vi "PicowattAVS47_Check_Queue.vi"(7 "error in (no error)":errorcluster caption="Fehler (Eingang, kein Fehler)", 10 "queue":refnum<queue>) -> (0 "error out":errorcluster caption="Fehler (Ausgang)", 1 "AVS47 Control Cluster":T1 {"AVS Excitation" items=["no Exc.", "3uV", "10uV", "30uV", "100uV", "300uV", "1mV", "3mV"]}, 3 "New Entries ?":bool)   [LabVIEW 2018]
uses:
  PicowattAVS47/AVS-Control-Cluster.ctl
panel:
  out "Numerisches Anzeigeelement":i32
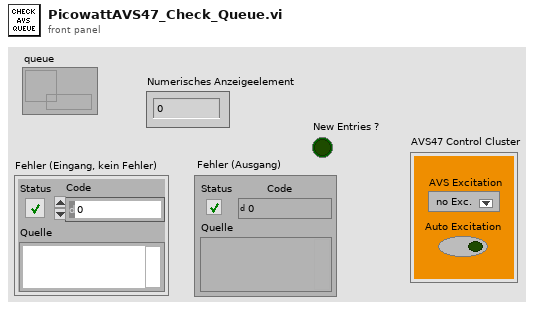
[diagram p1: front panel]
types:
  T1 = typedef "AVS-Control-Cluster.ctl" = cluster{"AVS Excitation":i16, "Auto Excitation":bool}
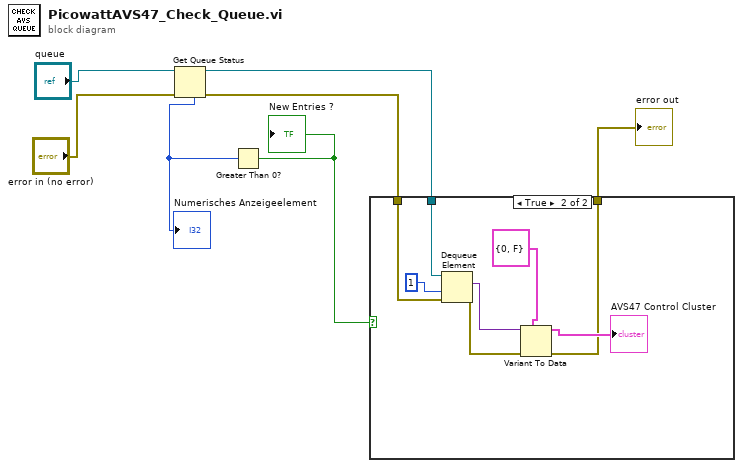
[diagram p0: block diagram]
diagram:
  n1 = Get Queue Status(queue="queue", error in (no error)="error in (no error)") -> (queue out=w3:refnum<queue>, error out=w2:errorcluster, # elements in queue=w5:i32)  [unwired: 1 in, 5 out]
  "Numerisches Anzeigeelement" <- w5
  n2 = Greater Than 0?(x=w5) -> (x > 0?=w4:bool)
  "New Entries ?" <- w4
  n3 = case shown="True" w4 {
    tunnel: w3 -> [_ w15]
    tunnel: w2 -> [w8 w16]
    tunnel: [w8 w9] -> w1
    frame False {
    }
    frame True {
      n4 = Dequeue Element(queue=w15, timeout in ms (-1)=1, error in (no error)=w16) -> (element=w13:variant, error out=w10:errorcluster)  [unwired: 2 out]
      n5 = Variant To Data(error in=w10, type=T1 {"AVS Excitation"=0, "Auto Excitation"=FALSE} ("AVS47 Control Cluster"), Variant=w13) -> (data=→"AVS47 Control Cluster":T1, error out=w9:errorcluster)
    }
  }
  "error out" <- w1
